vi "cRIO_FPGA_COMMUNICATION Zähler_Auslesen.vi"(0 "Station Index":T1) -> (14 "Zähler 1":u16, 15 "Zähler 1 == 0":bool, 16 "Zähler 2":u16, 17 "Zähler 2 == 0":bool, 18 "Zähler 3":u16, 19 "Zähler 3 == 0":bool)   [LabVIEW 2013, in "cRIO_FPGA_COMMUNICATION.lvlib"]
uses:
  cRIO_FPGA_COMMUNICATION.lvlib
  TYPES/TYPE Station Index.ctl
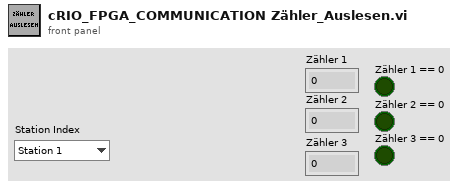
[diagram p1: front panel]
types:
  T1 = typedef "cRIO_FPGA_COMMUNICATION.lvlib/TYPE Station Index.ctl" = enum16{"Station 1", "Station 2", "Station 3", "Station 4", "Station 5", "Station 6", "Station 7", "Station 8", "Station 9", "Station 10", "Station 11", "Station 12", "Station 13", "Station 14", "Station 15", "Station 16", "Station 17", "Station 18", "Station 19", "Station 20"}
  T2 = enum16{"Init", "set Counter", "get Counter", "reset Counter", "configure Counter"}
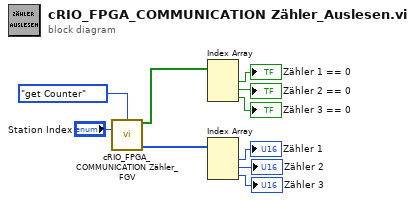
[diagram p0: block diagram]
diagram:
  n1 = call "cRIO_FPGA_COMMUNICATION Zähler_FGV.vi"("Set/Get/Configure"=T2."get Counter", "Station Index"="Station Index") -> ("ist Zähler == 0"=w4:bool[], "Zählerwerte"=w9:u16[])  [unwired: 12 in]
  n2 = Index Array(array=w4) -> (element #1=→"Zähler 1 == 0":bool, element #2=→"Zähler 2 == 0":bool, element #3=→"Zähler 3 == 0":bool)  [unwired: 3 in]
  n3 = Index Array(array=w9) -> (element #1=→"Zähler 1":u16, element #2=→"Zähler 2":u16, element #3=→"Zähler 3":u16)  [unwired: 3 in]
